vi "Translation2d_GetY.vi"(11 "In Translation":T1 {"Y" format="%14.3f"; "X" format="%14.3f"}) -> (3 "Y":dbl)   [LabVIEW 2019, in "Trajectory_Library.lvlib"]
doc: "Returns the Y component of the translation.\n\nParameters\n - IN Translation - This Translation data structure\n\nReturns:\n - Y- The Y component of the translation."
uses:
  Trajectory_Library.lvlib
  TypeDef/TRANSLATION2D.ctl
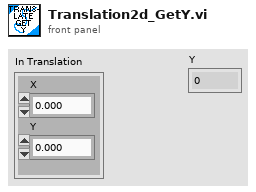
[diagram p1: front panel]
types:
  T1 = typedef "Trajectory_Library.lvlib/TRANSLATION2D.ctl" = cluster{"X":dbl, "Y":dbl}
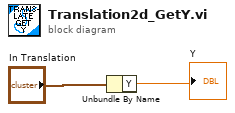
[diagram p0: block diagram]
diagram:
  n1 = Unbundle By Name("In Translation") -> ("Y"=→"Y":dbl)
